vi "Sans titre 8 (sous-VI).vi"(6 "Hexa en entrée":refnum<vi>, 7 "VOLTAGES Inputs":T1, 9 "Hexa 2 Used":refnum<vi>, 10 "Hexa 1":refnum<vi>, 11 "Boolean en entrée":refnum<vi>) -> (2 "Hexa 3":refnum<vi>, 3 "Boolean en sortie":refnum<vi>)   [LabVIEW 2015]
uses:
  controls/VOLTAGES_Inputs.ctl
  controls/HEXA_Inputs.ctl
  controls/QUAD_Inputs.ctl
panel:
  # "HEXAPOLE"
  # "QUADRIPOLE"
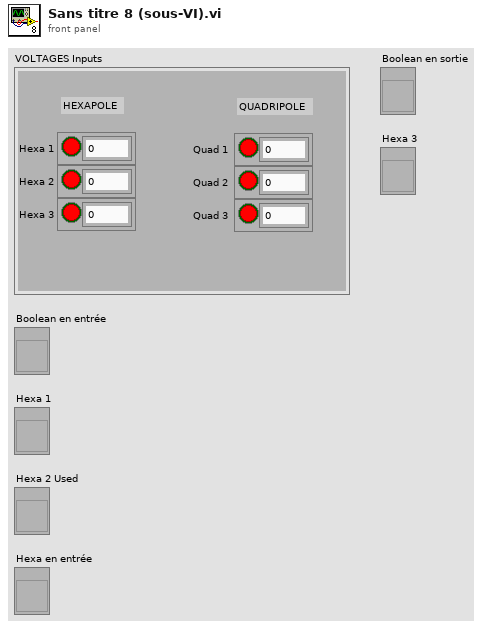
[diagram p1: front panel]
types:
  T1 = typedef "VOLTAGES_Inputs.ctl" = cluster{"Hexa 1":T2, "Hexa 2":T2, "Hexa 3":T2, "Quad 1":T3, "Quad 2":T3, "Quad 3":T3}
  T2 = typedef "HEXA_Inputs.ctl" = cluster{"Used":bool, "Voltage":dbl}
  T3 = typedef "QUAD_Inputs.ctl" = cluster{"Used":bool, "Voltage":dbl}
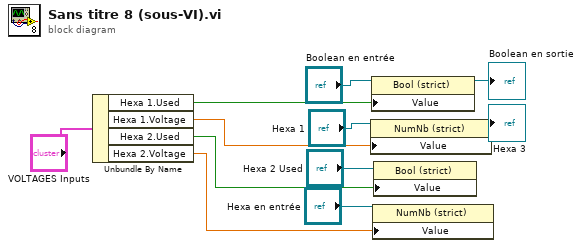
[diagram p0: block diagram]
diagram:
  n1 = Unbundle By Name("VOLTAGES Inputs") -> ("Hexa 1.Used"=w4:bool, "Hexa 1.Voltage"=w6:dbl, "Hexa 2.Used"=w10:bool, "Hexa 2.Voltage"=w11:dbl)
  n2 = property class="NumNb (strict)"(reference="Hexa 1", "Value"=w6) -> (reference out=→"Hexa 3":refnum<vi>)  [unwired: 1 in, 1 out]
  n3 = property class="Bool (strict)"(reference="Boolean en entrée", "Value"=w4) -> (reference out=→"Boolean en sortie":refnum<vi>)  [unwired: 1 in, 1 out]
  n4 = property class="NumNb (strict)"(reference="Hexa en entrée", "Value"=w11) -> ()  [unwired: 1 in, 2 out]
  n5 = property class="Bool (strict)"(reference="Hexa 2 Used", "Value"=w10) -> ()  [unwired: 1 in, 2 out]
